vi "FPGA_host_test.vi"() -> ()   [LabVIEW 2012]
doc: "This is an undocumented VI for testing the FPGA target (not maintained)."
uses:
  <vilib>/FPGAPlugInAG/PXI-7811R/niLvFpga_Open_PXI-7811R.vi
  <vilib>/Utility/error.llb/Error Cluster From Error Code.vi
  <vilib>/rvi/errors/niLvFpgaAdjustHostInterfaceError.vi
  <vilib>/FPGAPlugInAG/PXI-7811R/niLvFpga_Close_PXI-7811R.vi
  <vilib>/rvi/interface/nirviOpenFPGA/nirviOpenFPGA.xnode
  FPGA Bitfiles/NI-FPGA-PPG.lvproj_PXI-7811R_FPGA_target_main.vi.lvbitx
  <vilib>/rvi/interface/nirviMethod/nirviMethod.xnode
  <vilib>/rvi/interface/nirviReadWriteControl/nirviReadWriteControl.xnode
  <vilib>/rvi/interface/nirviCloseFPGA/nirviCloseFPGA.xnode
  <vilib>/FPGAPlugInAG/PXI-7811R/niLvFpga_WriteFifo_PXI-7811R.vi
  <vilib>/rvi/errors/niLvFpgaMergeErrorWithErrorCode.vi
  NiFpgaLv.dll
panel:
  in  "replace":bool
  in  "time":bool
  in  "mem_address":u32
  out "error out":errorcluster
  out "Empty Elements Remaining":u32
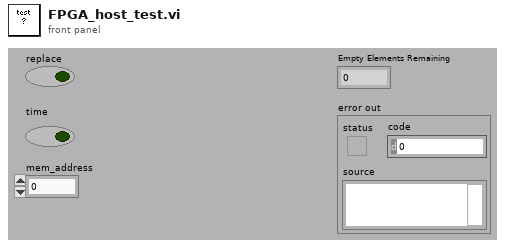
[diagram p1: front panel]
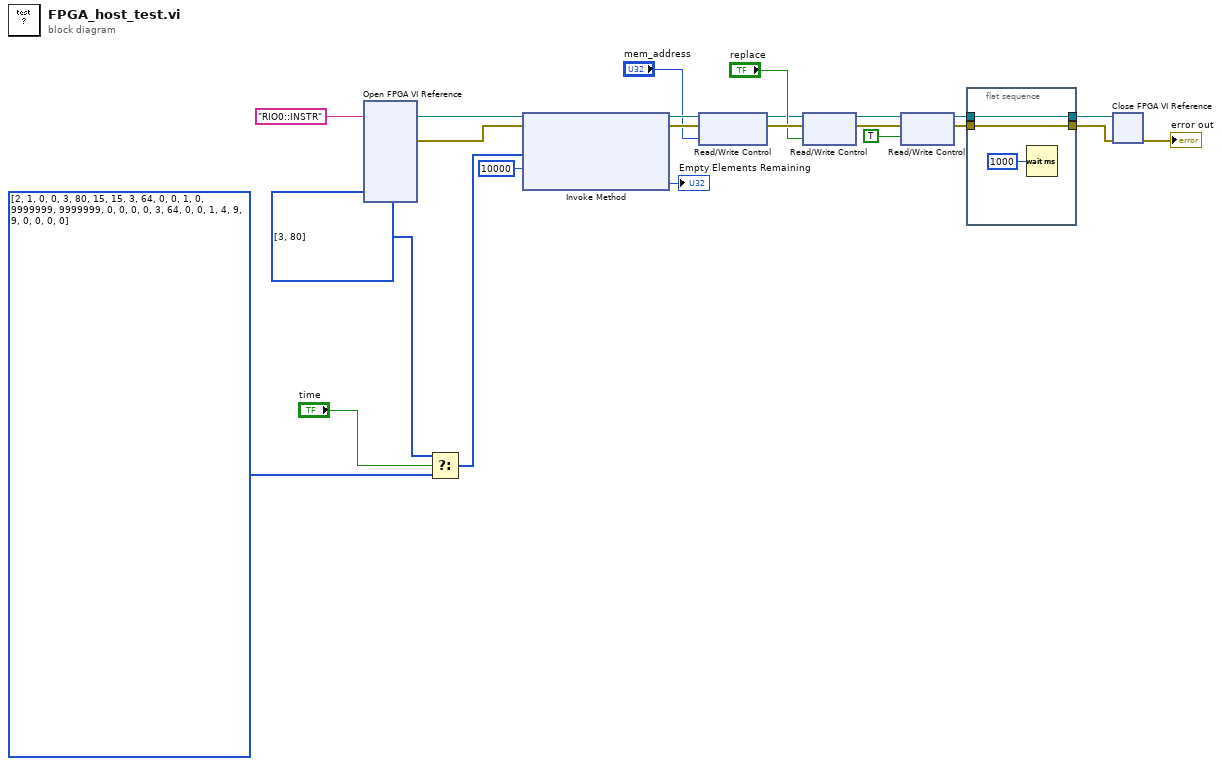
[diagram p0: block diagram]
diagram:
  # "7"
  # "6"
  # "5"
  # "4"
  # "3"
  # "2"
  # "1"
  n1 = xnode "Open FPGA VI Reference"("resource name"="RIO0::INSTR") -> ("FPGA VI Reference Out"=w3:refnum<k20>, "error out"=w19:errorcluster)  [unwired: 1 in]
  n2 = Select(t=u32[] [3, 80], s="time", f=u32[] [2, 1, 0, 0, 3, 80, 15, 15, 3, 64, 0, 0, 1, 0, 9999999, 9999999, 0, 0, 0, 0, 3, 64, 0, 0, 1, 4, 9, 9, 0, 0, 0, 0]) -> (s? t:f=w5:u32[])
  n3 = xnode "Invoke Method"("FPGA VI Reference In"=w3, "error in"=w19, "Data"=w5, "Timeout (ms)"=10000) -> ("FPGA VI Reference Out"=w13:refnum<k20>, "error out"=w12:errorcluster, "Empty Elements Remaining"=→"Empty Elements Remaining":u32)
  n4 = xnode "Read/Write Control"("FPGA VI Reference In"=w13, "error in"=w12, "mem_addr"="mem_address") -> ("FPGA VI Reference Out"=w6:refnum<k20>, "error out"=w8:errorcluster)
  n5 = xnode "Read/Write Control"("FPGA VI Reference In"=w6, "error in"=w8, "replace"="replace") -> ("FPGA VI Reference Out"=w9:refnum<k20>, "error out"=w10:errorcluster)
  n6 = xnode "Read/Write Control"("FPGA VI Reference In"=w9, "error in"=w10, "load"=TRUE) -> ("FPGA VI Reference Out"=w16:refnum<k20>, "error out"=w15:errorcluster)
  n7 = flat-sequence {
    tunnel: w16 -> [w25]
    tunnel: w15 -> [w24]
    tunnel: [w25] -> w2
    tunnel: [w24] -> w1
    frame #0 {
      n8 = Wait (ms)(milliseconds to wait=u32 1000) -> ()  [unwired: 1 out]
    }
  }
  n9 = xnode "Close FPGA VI Reference"("FPGA VI Reference In"=w2, "error in"=w1) -> ("error out"=→"error out":errorcluster)
